vi "Sensor_Console.vi"(8 "error in":errorcluster) -> (0 "error out":errorcluster)   [LabVIEW 2013, in "Sensor Console.lvlib"]
doc: "This is the sensor interface module (a free running module of the ATM simulator). \n\nIt is closed using a user event. It communicates with the other modules using a queue based API which has comms modules that can be swapped if required."
uses:
  Sensor Console.lvlib
  Private Controls/Sensor Data Cluster.ctl
  Private Controls/Sensor Action.ctl
  User Events/Controls/UE Abort Action.ctl
  Controller/Contoller.lvlib
  Error Handler/Error Handler.lvlib
panel:
  in  "Deposit Recieved":bool
  in  "Funds Disbursed":bool
  # "[Covers: UI4]"
  # "[Covers: UI4A]"
  # "[Covers: UI4B]"
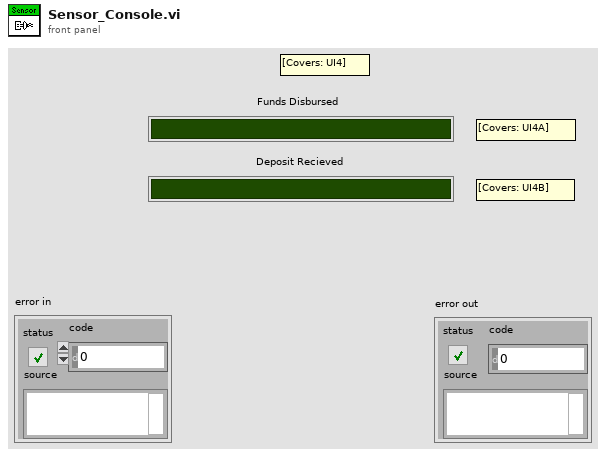
[diagram p1: front panel]
types:
  T1 = typedef "Sensor Console.lvlib/Sensor Data Cluster.ctl" = cluster{"Data":variant, "Action":T2}
  T2 = typedef "Sensor Console.lvlib/Sensor Action.ctl" = enum16{"Init", "Deposit", "Disburse", "Error", "Exit"}
  T3 = typedef "UE Abort Action.ctl" = enum16{"Destroy", "Get", "Create"}
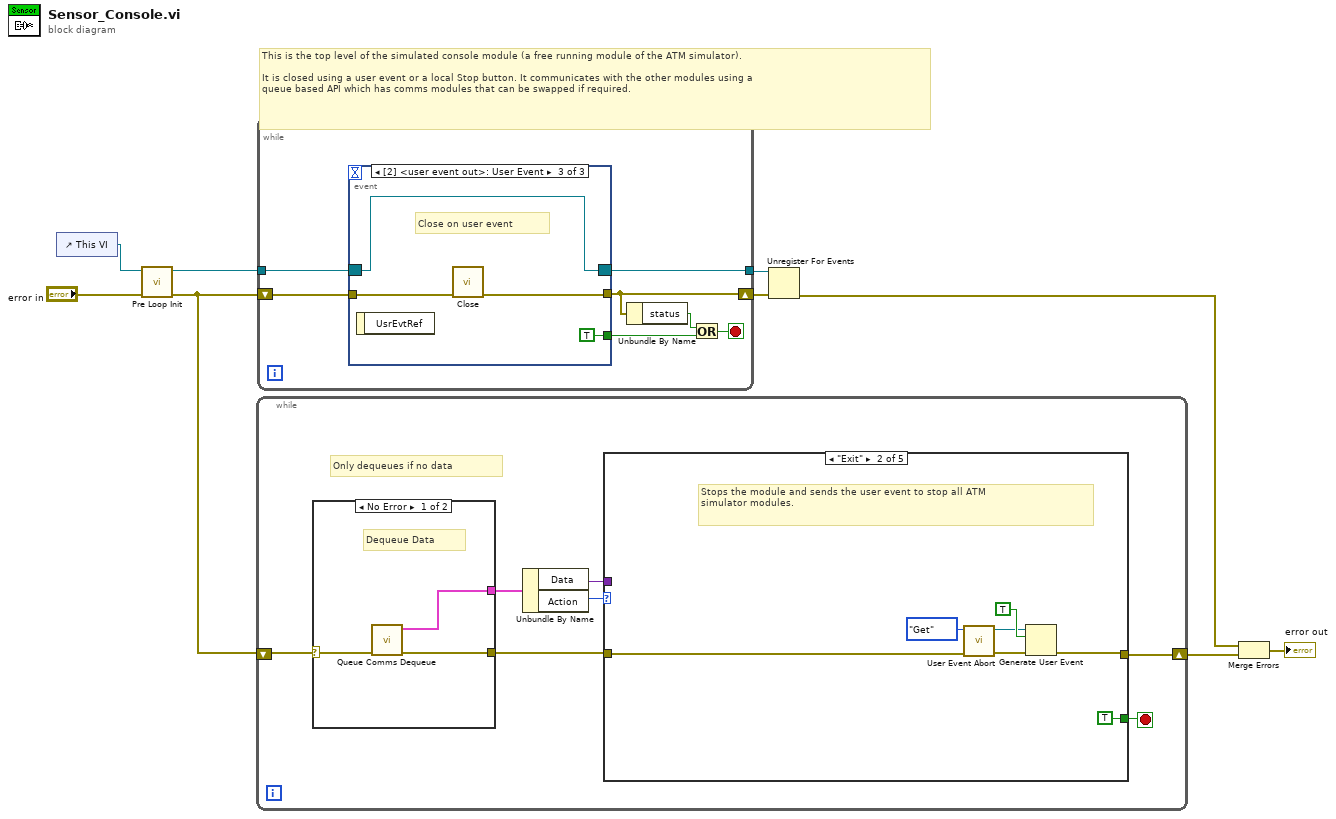
[diagram p0: block diagram]
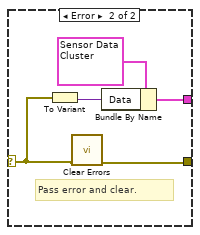
[diagram p2: hidden frame]
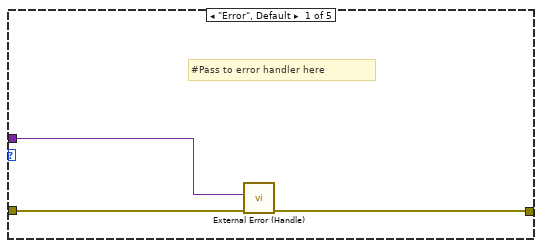
[diagram p3: hidden frame]
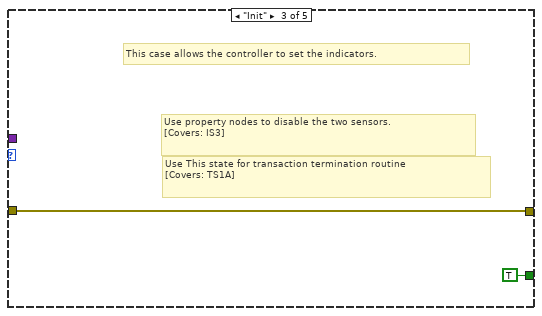
[diagram p4: hidden frame]
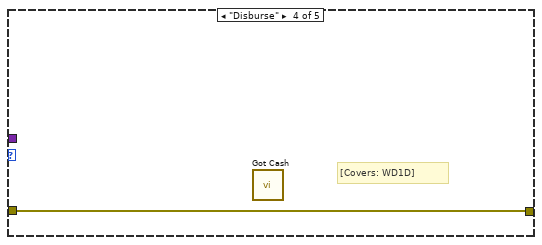
[diagram p5: hidden frame]
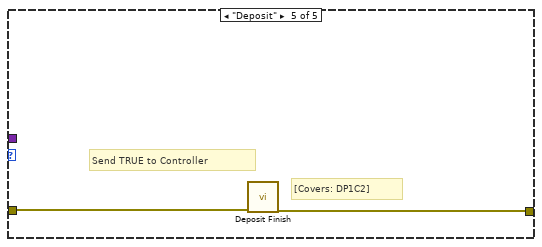
[diagram p6: hidden frame]
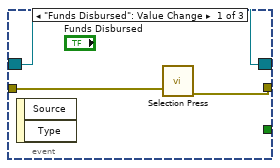
[diagram p7: hidden frame]
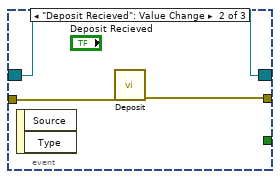
[diagram p8: hidden frame]
diagram:
  # "This is the top level of the simulated console module (a free running module of the ATM simulator). \n\nIt is closed using a user event or a local Stop button. It communicates with the other modules using a\nqueue based API which has comms modules that can be swapped if required."
  n1 = control-ref of="This VI"() -> (w9:refnum<vi>)
  n2 = call "Pre Loop Init.vi"("error in"="error in", "Ref In"=w9) -> ("error out"=w4:errorcluster, "Event Registration Refnum"=w7:refnum<event-registration>)  [unwired: 8 in]
  n3 = while {
    shift-right: [w10] -> w2
    shift-left: w4 -> [w15]
    stop <- w16 stop-if-true
    # "Only dequeues if no data"
    n4 = case shown="No Error" w15 {
      selector: w15 -> [w18 w21]
      tunnel: [w19 w20] -> w13
      tunnel: [w17 w22] -> w14
      frame No Error {
        # "Dequeue Data"
        n5 = call "Queue Comms Dequeue.vi"("error in"=w18) -> ("error out"=w19:errorcluster, "Data Out"=w17:T1)  [unwired: 9 in]
      }
      frame Error {
        # "Pass error and clear."
        n6 = To Variant(anything=w21) -> (Variant=w23:variant)
        n7 = call <vilib>:"Clear Errors.vi"("error in (no error)"=w21) -> ("error out"=w20:errorcluster)  [unwired: 6 in]
        n8 = Bundle By Name(cluster=T1 {"Data"=variant, "Action"=enum."Error"} ("Cluster"), "Data"=w23) -> (w22:T1)
      }
    }
    n9 = Unbundle By Name(w14) -> ("Data"=w11:variant, "Action"=w12:T2)
    n10 = case shown="\"Exit\"" w12 {
      tunnel: [_ TRUE TRUE _ _] -> w16
      tunnel: w13 -> [w27 w29 w35 w37 w39]
      tunnel: w11 -> [w25 _ _ _ _]
      tunnel: [w26 w28 w35 w37 w38] -> w10
      frame "Error", Default {
        # "#Pass to error handler here"
        n11 = call "External Error (Handle).vi"("error in"=w27, "Data"=w25) -> ("error out"=w26:errorcluster)  [unwired: 9 in]
      }
      frame "Exit" {
        # "Stops the module and sends the user event to stop all ATM\nsimulator modules."
        n12 = call "User Event Abort.vi"("error in"=w29, "Action"=UE_Abort_Action."Get") -> ("error out"=w31:errorcluster, "user event out"=w32:refnum<user-event>)  [unwired: 8 in]
        n13 = Generate User Event(user event=w32, event data cluster=TRUE ("event data"), error in=w31) -> (error out=w28:errorcluster)  [unwired: 1 in, 1 out]
      }
      frame "Init" {
        # "Use This state for transaction termination routine\n[Covers: TS1A]"
        # "Use property nodes to disable the two sensors.\n[Covers: IS3]"
        # "This case allows the controller to set the indicators."
      }
      frame "Disburse" {
        # "[Covers: WD1D]"
        n14 = call "Got Cash.vi"() -> ()  [unwired: 11 in, 1 out]
      }
      frame "Deposit" {
        # "[Covers: DP1C2]"
        # "Send TRUE to Controller"
        n15 = call "Deposit Finish.vi"("error in"=w39) -> ("error out"=w38:errorcluster)  [unwired: 10 in]
      }
    }
  }
  n16 = while {
    shift-right: [w43] -> w6
    shift-left: w4 -> [w46]
    tunnel: w7 -> [w41]
    tunnel: [w40] -> w5
    stop <- w44 stop-if-true
    n17 = event shown="[2] <user event out>: User Event" {
      selector: w41 -> [w49 w52 w56]
      dyn-events: [w49 w52 w56] -> w40
      timeout: _ -> [_ _ _]
      tunnel: w46 -> [w48 w51 w55]
      tunnel: [w47 w50 w54] -> w43
      tunnel: [_ _ TRUE ("stop")] -> w45
      event "Funds Disbursed": Value Change {
        n18 = event-data() -> ()  [unwired: 1 in, 2 out]
        n19 = call "Selection Press.vi"("error in"=w48) -> ("error out"=w47:errorcluster)  [unwired: 10 in]
      }
      event "Deposit Recieved": Value Change {
        n20 = event-data() -> ()  [unwired: 1 in, 2 out]
        n21 = call "Deposit.vi"("error in"=w51) -> ("error out"=w50:errorcluster)  [unwired: 10 in]
      }
      event User Event {
        # "Close on user event"
        n22 = event-data() -> ()  [unwired: 1 in, 1 out]
        n23 = call "Close.vi"("error in"=w55) -> ("error out"=w54:errorcluster)  [unwired: 10 in]
      }
    }
    n24 = Unbundle By Name(w43) -> ("status"=w42:bool)
    n25 = Or(x=w42, y=w45) -> (x .or. y?=w44:bool)
  }
  n26 = Unregister For Events(event registration refnum=w5, error in=w6) -> (error out=w1:errorcluster)
  n27 = Merge Errors(w1, w2) -> (→"error out":errorcluster)
